vi "Read absolute position.vi"(4 "error in (no error)":errorcluster, 6 "Axis (1)":i32=1 min=1 max=3, 7 "VISA resource name":refnum<visa-resource-name>) -> (0 "error out":errorcluster, 2 "Position (units)":dbl format="%.6g", 3 "VISA resource name out":refnum<visa-resource-name>)   [LabVIEW 2019, in "Newport ESP301.lvlib"]
doc: "Reports actual position."
uses:
  Newport ESP301.lvlib
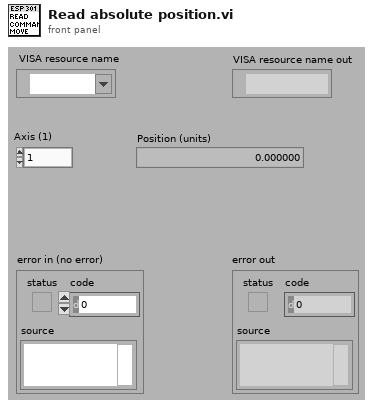
[diagram p1: front panel]
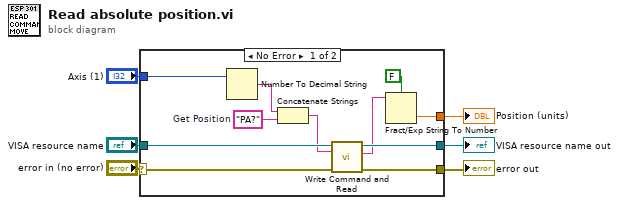
[diagram p0: block diagram]
diagram:
  n1 = case shown="No Error" "error in (no error)" {
    selector: "error in (no error)" -> [w12 w19]
    tunnel: [w16 w19] -> w6
    tunnel: "VISA resource name" -> [w17 w18]
    tunnel: [w15 w18] -> w5
    tunnel: [w13 _] -> w3
    tunnel: "Axis (1)" -> [w8 _]
    frame No Error {
      w11 = "PA?"  # Get Position
      n2 = Number To Decimal String(number=w8) -> (decimal integer string=w10:string)  [unwired: 1 in]
      n3 = Concatenate Strings(w10, w11) -> (w9:string)
      n4 = call "Write Command and Read.vi"("error in (no error)"=w12, "Command"=w9, "VISA resource name"=w17) -> ("error out"=w16:errorcluster, "Returned string"=w14:string, "VISA resource name out"=w15:refnum<visa-resource-name>)  [unwired: 4 in]
      n5 = Fract/Exp String To Number(use system decimal point (T)=FALSE ("utiliser le séparateur décimal du système (V)"), string=w14) -> (number=w13:dbl)  [unwired: 2 in, 1 out]
    }
    frame Error {
    }
  }
  "error out" <- w6
  "VISA resource name out" <- w5
  "Position (units)" <- w3
